vi "Cents2DollarString-Main.vi"() -> ()   [LabVIEW 2019]
panel:
  out "Dollars":string
  in  "Cents":dbl
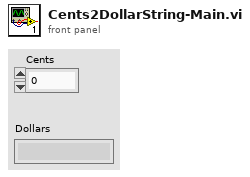
[diagram p1: front panel]
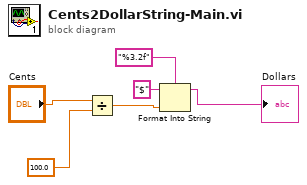
[diagram p0: block diagram]
diagram:
  n1 = Divide(x="Cents", y=100.0) -> (x/y=w4:dbl)
  n2 = Format Into String(format string="%3.2f", initial string="$", w4) -> (resulting string=→"Dollars":string)  [unwired: 1 in, 1 out]
